vi "Ensure qwtb_info exist.vi"(8 "error in":errorcluster, 11 "Measurement path":path) -> (0 "error out":errorcluster)   [LabVIEW 2020]
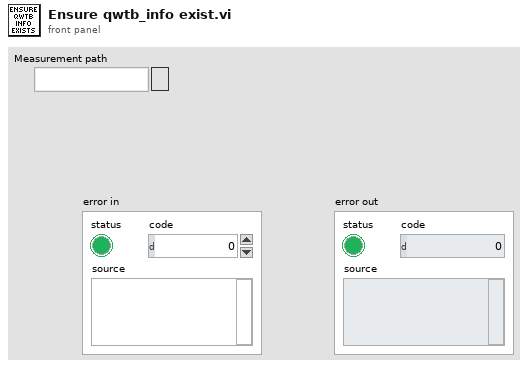
[diagram p1: front panel]
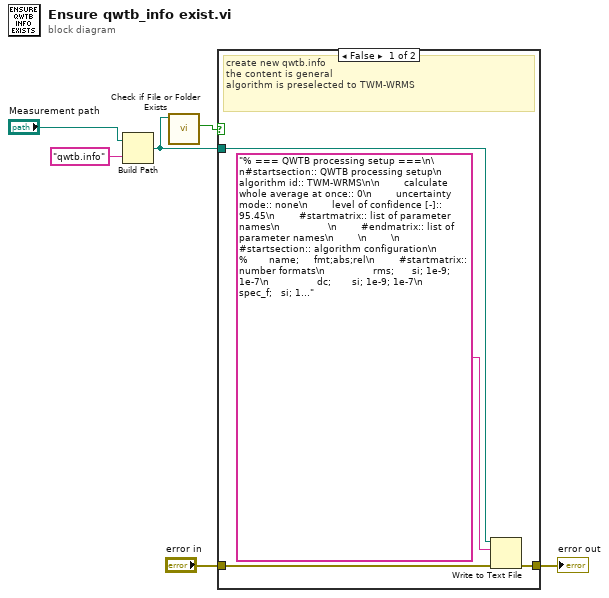
[diagram p0: block diagram]
diagram:
  n1 = Build Path(base path="Measurement path", name or relative path="qwtb.info") -> (appended path=w3:path)
  n2 = call <vilib>:"Check if File or Folder Exists.vi"("path"=w3) -> ("file or folder exists?"=w4:bool)  [unwired: 8 in, 2 out]
  n3 = case shown="False" w4 {
    tunnel: w3 -> [w9 _]
    tunnel: "error in" -> [w8 w11]
    tunnel: [w7 w11] -> w1
    frame False {
      # "create new qwtb.info\nthe content is general\nalgorithm is preselected to TWM-WRMS"
      n4 = Write to Text File(file (use dialog)=w9, text="% === QWTB processing setup ===\n\n#startsection:: QWTB processing setup\n        algorithm id:: TWM-WRMS\n\n        calculate whole average at once:: 0\n        uncertainty mode:: none\n        level of confidence [-]:: 95.45\n        #startmatrix:: list of parameter names\n                \n        #endmatrix:: list of parameter names\n        \n        \n        #startsection:: algorithm configuration\n                        %       name;     fmt;abs;rel\n        #startmatrix:: number formats\n                rms;      si; 1e-9; 1e-7\n                dc;       si; 1e-9; 1e-7\n                spec_f;   si; 1e-9; 1e-7\n                spec_A;   si; 1e-9; 1e-7\n        #endmatrix:: number formats\n        #startmatrix:: graphs\n\t\tspec_f; spec_A\n        #endmatrix:: graphs\n        spectrum:: spec_A\n        #endsection:: algorithm configuration\n#endsection:: QWTB processing setup", error in=w8) -> (error out=w7:errorcluster)  [unwired: 1 in, 2 out]
    }
    frame True {
      # "qwtb.info already exist, nothing to do"
    }
  }
  "error out" <- w1
